vi "Postion Update.vi"(2 "Y position in":dbl, 3 "X position in":dbl, 4 "Distance":dbl, 5 "Heading":dbl) -> (0 "Y position":dbl, 1 "X position":dbl)   [LabVIEW 2018]
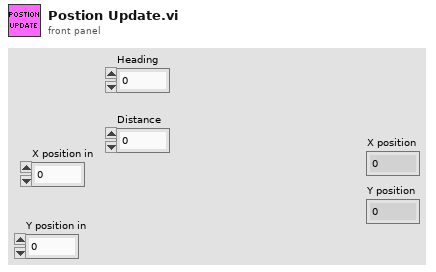
[diagram p1: front panel]
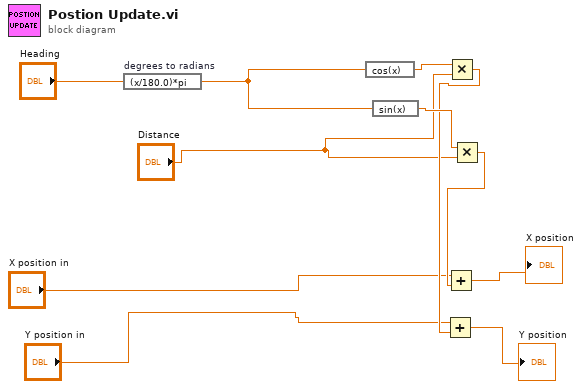
[diagram p0: block diagram]
diagram:
  n1 = expression code="(x/180.0)*pi" "degrees to radians"("Heading") -> (w5:dbl)
  n2 = expression code="cos(x)"(w5) -> (w10:dbl)
  n3 = expression code="sin(x)"(w5) -> (w11:dbl)
  n4 = Multiply(x=w10, y="Distance") -> (x*y=w8:dbl)
  n5 = Add(x="Y position in", y=w8) -> (x+y=→"Y position":dbl)
  n6 = Multiply(x=w11, y="Distance") -> (x*y=w9:dbl)
  n7 = Add(x="X position in", y=w9) -> (x+y=→"X position":dbl)
